vi "FlexDDS-NG_time_to_MP.vi"(9 "sweep time tolerance (us)":dbl, 10 "freq_diff (Hz)":dbl, 11 "sweep time (ms)":dbl) -> (1 "Dt (s)":dbl, 2 "ctr":i32, 3 "Df (Hz)":dbl, 4 "T (in  s)":dbl, 5 "P":u16, 6 "num":dbl, 7 "M":i32)   [LabVIEW 2010]
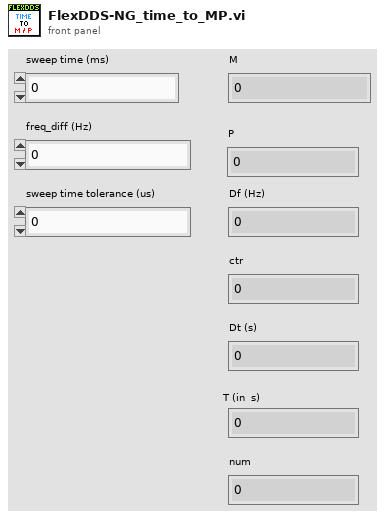
[diagram p1: front panel]
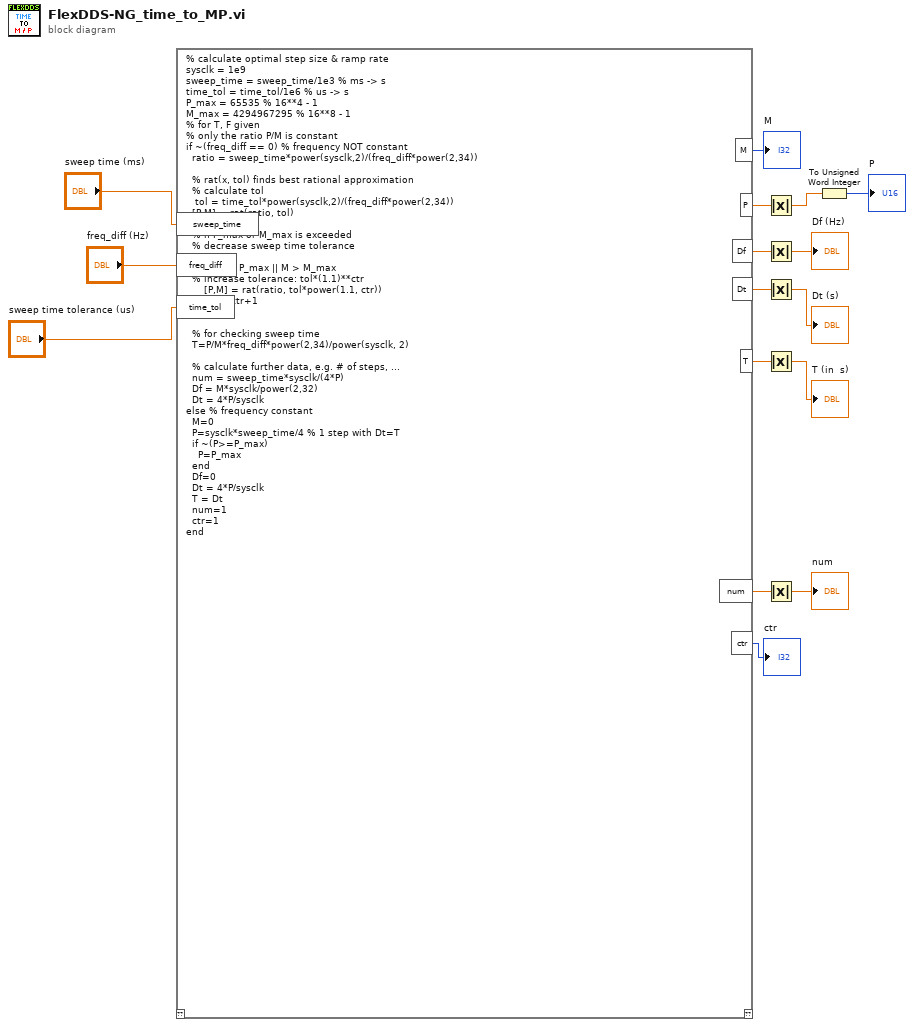
[diagram p0: block diagram]
diagram:
  n1 = mathscript code="% calculate optimal step size & ramp rate\nsysclk = 1e9\nsweep_time = sweep_time/1e3 % ms -> s\ntime_tol = time_tol/1e6 % us -> s\nP_max = 65535 % 16**4 - 1\nM_max = 4294967295 % 16**8 - 1\n% for T, F given\n% only the ratio P/M is constant\nif ~(freq_diff == 0) % frequency NOT constant\n  ratio = sweep_time*power(sysclk,2)/(freq_diff*power(2,34))\n\n  % rat(x, tol) finds best rational approximation\n  % calculate tol\n   tol = time_tol*power(sysclk,2)/(freq_diff*power(2,34))\n  [P,M] = rat(ratio, tol)\n\n  % if P_max or M_max is exceeded\n  % decrease sweep time tolerance\n  ctr = 1\n  while P > P_max || M > M_max\n  % increase tolerance: tol*(1.1)**ctr\n      [P,M] = rat(ratio, tol*power(1.1, ctr))\n      ctr = ctr+1\n  end\n\n  % for checking sweep time\n  T=P/M*freq_diff*power(2,34)/power(sysclk, 2)\n\n  % calculate further data, e.g. # of steps, ...\n  num = sweep_time*sysclk/(4*P)\n  Df = M*sysclk/power(2,32)\n  Dt = 4*P/sysclk\nelse % frequency constant\n  M=0\n  P=sysclk*sweep_time/4 % 1 step with Dt=T\n  if ~(P>=P_max)\n    P=P_max\n  end\n  Df=0\n  Dt = 4*P/sysclk\n  T = Dt\n  num=1\n  ctr=1\nend"("sweep_time"="sweep time (ms)", "freq_diff"="freq_diff (Hz)", "time_tol"="sweep time tolerance (us)") -> ("M"=→"M":i32, "P"=w11:cdb, "T"=w6:cdb, "Df"=w10:cdb, "Dt"=w8:cdb, "ctr"=→"ctr":i32, "num"=w4:cdb)  [unwired: 1 in, 1 out]
  n2 = Absolute Value(x=w11) -> (abs(x)=w2:dbl)
  n3 = Absolute Value(x=w10) -> (abs(x)=→"Df (Hz)":dbl)
  n4 = Absolute Value(x=w8) -> (abs(x)=→"Dt (s)":dbl)
  n5 = Absolute Value(x=w6) -> (abs(x)=→"T (in  s)":dbl)
  n6 = Absolute Value(x=w4) -> (abs(x)=→"num":dbl)
  n7 = To Unsigned Word Integer(number=w2) -> (unsigned 16bit integer=→"P":u16)
